vi "SwissSPAD Live_Get SS2 Gate Configuration Name.vi"(9 "Gate Configuration Definition in":T1, 11 "Gate Configurations Definitions":T1[](array[typedef])) -> (0 "Gate Configuration Found?":bool, 1 "Configuration ID":i32, 2 "Gate Definition Found?":bool, 3 "Gate Configuration Name":string)   [LabVIEW 2021]
uses:
  SwissSPAD Live_SS2 Gate Configuration.ctl
  SwissSPAD Live_SS2 Gate Definition.ctl
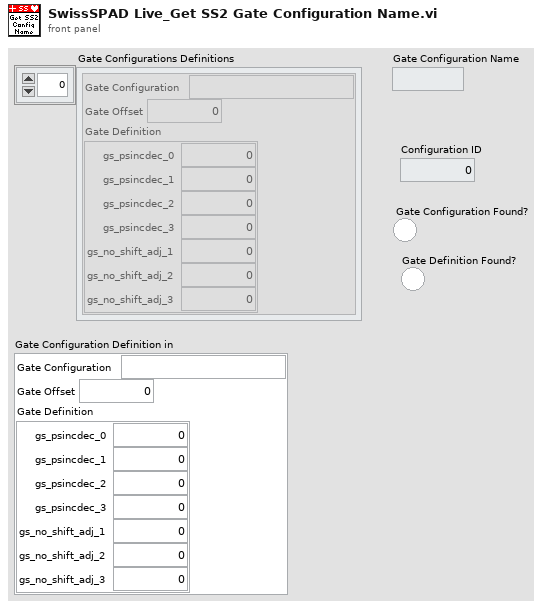
[diagram p1: front panel]
types:
  T1 = typedef "SwissSPAD Live_SS2 Gate Configuration.ctl" = cluster{"Gate Configuration":string, "Gate Offset":u32, "Gate Definition":T2}
  T2 = typedef "SwissSPAD Live_SS2 Gate Definition.ctl" = cluster{"gs_psincdec_0":u32, "gs_psincdec_1":u32, "gs_psincdec_2":u32, "gs_psincdec_3":u32, "gs_no_shift_adj_1":u32, "gs_no_shift_adj_2":u32, "gs_no_shift_adj_3":u32}
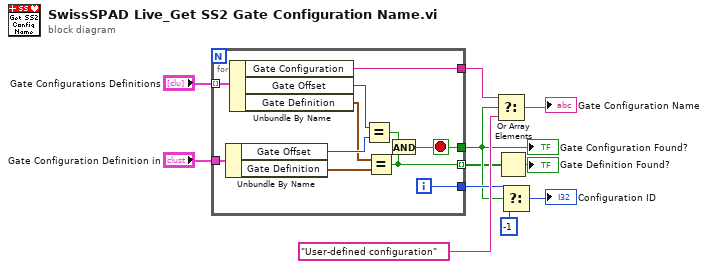
[diagram p0: block diagram]
diagram:
  n1 = for {
    tunnel: "Gate Configurations Definitions" -> [w15] mode=indexing
    tunnel: [w16] -> w5
    tunnel: "Gate Configuration Definition in" -> [w22]
    tunnel: [w14] -> w9
    tunnel: [w13] -> w6
    tunnel: [w12] -> w2 mode=indexing
    i -> [w13]
    stop <- w16 stop-if-true
    n2 = Unbundle By Name(w22) -> ("Gate Offset"=w20:u32, "Gate Definition"=w18:T2)
    n3 = Unbundle By Name(w15) -> ("Gate Configuration"=w14:string, "Gate Offset"=w21:u32, "Gate Definition"=w19:T2)
    n4 = Equal?(x=w21, y=w20) -> (x = y?=w17:bool)
    n5 = Equal?(x=w19, y=w18) -> (x = y?=w12:bool)
    n6 = And(x=w17, y=w12) -> (x .and. y?=w16:bool)
  }
  "Gate Configuration Found?" <- w5
  n7 = Select(t=w9, s=w5, f="User-defined configuration") -> (s? t:f=→"Gate Configuration Name":string)
  n8 = Or Array Elements(Boolean array=w2) -> (logical OR=→"Gate Definition Found?":bool)
  n9 = Select(t=w6, s=w5, f=-1) -> (s? t:f=→"Configuration ID":i32)
